vi "Get Object Metadata.vi"(6 "Version ID":string, 7 "Request Parameters":T1, 8 "error in (no error)":errorcluster, 9 "Bucket":string, 10 "Path":string) -> (0 "error out":errorcluster, 2 "HeadObjectResult":T3)   [LabVIEW 2011, in "LV Interface for Amazon S3.lvlib"]
doc: "This operation <B>retrieves information and metadata associated with an object</B> from Amazon S3. You <B>must have READ access</B> to the object. If you grant READ access to the anonymous user, you can return the object without using an authorization header."
uses:
  LV Interface for Amazon S3.lvlib
  Typedefs/AMZ_S3_API_HEADObjectResult.ctl
  Typedefs/AMZ_S3_API_GETObjectResult.ctl
  Typedefs/AMZ_S3_Key-Value pair.ctl
  Typedefs/AMZ_S3_API_GET Object Request Parameters.ctl
  Typedefs/AMZ_S3_API_GET Request Range.ctl
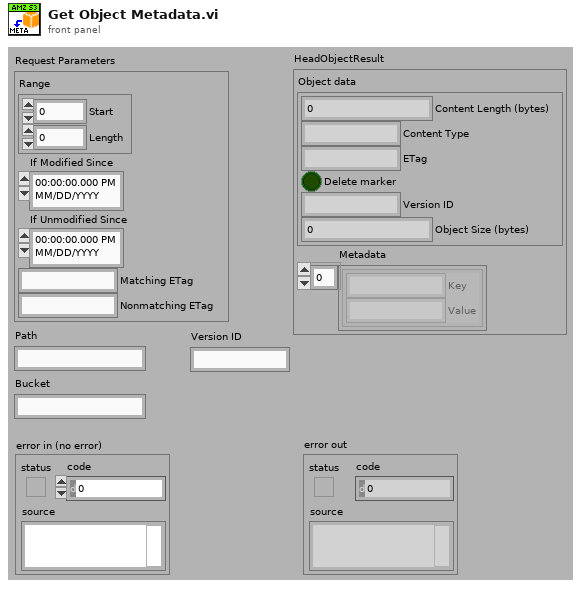
[diagram p1: front panel]
types:
  T1 = typedef "LV Interface for Amazon S3.lvlib/AMZ_S3_API_GET Object Request Parameters.ctl" = cluster{"Range":T2, "If Modified Since":timestamp, "If Unmodified Since":timestamp, "Matching ETag":string, "Nonmatching ETag":string}
  T2 = typedef "LV Interface for Amazon S3.lvlib/AMZ_S3_API_GET Request Range.ctl" = cluster{"Start":i64, "Length":i64}
  T3 = typedef "LV Interface for Amazon S3.lvlib/AMZ_S3_API_HEADObjectResult.ctl" = cluster{"Object data":T4, "Metadata":T5[]}
  T4 = typedef "LV Interface for Amazon S3.lvlib/AMZ_S3_API_GETObjectResult.ctl" = cluster{"Content Length (bytes)":u64, "Content Type":string, "ETag":string, "Delete marker":bool, "Version ID":string, "Object Size (bytes)":u64}
  T5 = typedef "LV Interface for Amazon S3.lvlib/AMZ_S3_Key-Value pair.ctl" = cluster{"Key":string, "Value":string}
  T6 = typedef "LV Interface for Amazon S3.lvlib/AMZ_S3_HTTP Header-Value pair.ctl" = cluster{"Header":string, "Value":string}
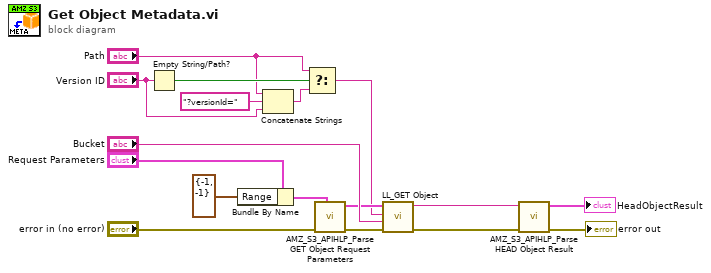
[diagram p0: block diagram]
diagram:
  n1 = Empty String/Path?(string/path="Version ID") -> (empty?=w13:bool)
  n2 = Bundle By Name(cluster="Request Parameters", "Range"=T2 {"Start"=-1, "Length"=-1}) -> (w1:T1)
  n3 = Concatenate Strings("Path", "?versionId=" ("string"), "Version ID") -> (w9:string)
  n4 = Select(t="Path", s=w13, f=w9) -> (s? t:f=w8:string)
  n5 = call "AMZ_S3_APIHLP_Parse GET Object Request Parameters.vi"("GET Object Request Parameters"=w1, "error in (no error)"="error in (no error)") -> ("error out"=w16:errorcluster, "HTTP Headers"=w15:T6[])  [unwired: 8 in]
  n6 = call "LL_GET Object.vi"("error in (no error)"=w16, "Bucket"="Bucket", "Path and query string"=w8, "Headers"=w15) -> ("error out"=w7:errorcluster, "Response header"=w6:string)  [unwired: 4 in, 2 out]
  n7 = call "AMZ_S3_APIHLP_Parse HEAD Object Result.vi"("error in (no error)"=w7, "Response header"=w6) -> ("error out"=→"error out":errorcluster, "HeadObjectResult"=→"HeadObjectResult":T3)  [unwired: 8 in]
